vi "Plotting Assemble.vi"(4 "Custom Titles":string[](array[string])=["System Date", "System Time", "Elapsed Time (sec)", "Elapsed Time (hrs)", "Voltage (V)", "RMS Current (Amps)", "Power (Watts)", "Watt Hours (Wh)", "Voltage Total Harmonic Distortion (%)", "Frequency (Hz)", "Apparent Power (VA)", "Power Factor", "TC 1", "TC 2", "TC 3", "TC 4", "TC 5", "TC 6", "TC 7", "TC 8", "TC 9", "TC 10", "TC 11", "TC 12", "TC 13", "TC 14", "TC 15", "TC 16", "TC 17", "TC 18", "TC 19", "TC 20", "TC 21", "TC 22", "TC 23", "TC 24", "TC 25", "TC 26", "TC 27", "TC 28", "TC 29", "TC 30", "AUX 1", "AUX 2", "CAL CL", "Room Setpoint Temperature", "Room Setpoint Humidity", "Room Temperature (°F)", "Room Humidity (%)", "Door Enable", "Room Setpoint Cool Temperature", "Room Setpoint Dehumidification Temperature", "Supply Temperature (°F)", "Cool Temperature (°F)", "Dehumidification Temperature (°F)", "Glycol Temperature (°F)", "Heat Rate (%)", "Steam Rate (%)", "Cool Rate (%)", "Dehumidification Rate (%)", "Room Status", "Room Dry P", "Room Dry I", "Room Humidity P", "Room Humidity I", "Room Heat P", "Room Heat I", "Room Cool Temperature P", "Room Cool Temperature I", "Room Dehumidification Temperature P", "Room Dehumidification Temperature I", "Voltage Setpoint 1", "60 Hz Power", "50 Hz Power", "120V Range", "240V Range", "Ground Line", "Ground Neutral", "Measure Ground Leakage Current", "Room OK", "S1 Freezer Relay", "S1 Cab Relay", "S1 Slide Relay", "Recording Data", "CVS Location", "Point Location"], 6 "Listbox Item Names":string[](array[string])=["System Date", "System Time", "Elapsed Time (sec)", "Elapsed Time (hrs)", "Voltage (V)", "RMS Current (Amps)", "Power (Watts)", "Watt Hours (Wh)", "Voltage Total Harmonic Distortion (%)", "Frequency (Hz)", "Apparent Power (VA)", "Power Factor", "TC 1", "TC 2", "TC 3", "TC 4", "TC 5", "TC 6", "TC 7", "TC 8", "TC 9", "TC 10", "TC 11", "TC 12", "TC 13", "TC 14", "TC 15", "TC 16", "TC 17", "TC 18", "TC 19", "TC 20", "TC 21", "TC 22", "TC 23", "TC 24", "TC 25", "TC 26", "TC 27", "TC 28", "TC 29", "TC 30", "AUX 1", "AUX 2", "CAL CL", "Room Setpoint Temperature", "Room Setpoint Humidity", "Room Temperature (°F)", "Room Humidity (%)", "Door Enable", "Room Setpoint Cool Temperature", "Room Setpoint Dehumidification Temperature", "Supply Temperature (°F)", "Cool Temperature (°F)", "Dehumidification Temperature (°F)", "Glycol Temperature (°F)", "Heat Rate (%)", "Steam Rate (%)", "Cool Rate (%)", "Dehumidification Rate (%)", "Room Status", "Room Dry P", "Room Dry I", "Room Humidity P", "Room Humidity I", "Room Heat P", "Room Heat I", "Room Cool Temperature P", "Room Cool Temperature I", "Room Dehumidification Temperature P", "Room Dehumidification Temperature I", "Voltage Setpoint 1", "60 Hz Power", "50 Hz Power", "120V Range", "240V Range", "Ground Line", "Ground Neutral", "Measure Ground Leakage Current", "Room OK", "S1 Freezer Relay", "S1 Cab Relay", "S1 Slide Relay", "Recording Data", "CVS Location", "Point Location"], 7 "Use Filter?":bool, 8 "Error In":errorcluster, 9 "Full Item Names":string[](array[string])=["System Date", "System Time", "Elapsed Time (sec)", "Elapsed Time (hrs)", "Voltage (V)", "RMS Current (Amps)", "Power (Watts)", "Watt Hours (Wh)", "Voltage Total Harmonic Distortion (%)", "Frequency (Hz)", "Apparent Power (VA)", "Power Factor", "TC 1", "TC 2", "TC 3", "TC 4", "TC 5", "TC 6", "TC 7", "TC 8", "TC 9", "TC 10", "TC 11", "TC 12", "TC 13", "TC 14", "TC 15", "TC 16", "TC 17", "TC 18", "TC 19", "TC 20", "TC 21", "TC 22", "TC 23", "TC 24", "TC 25", "TC 26", "TC 27", "TC 28", "TC 29", "TC 30", "AUX 1", "AUX 2", "CAL CL", "Room Setpoint Temperature", "Room Setpoint Humidity", "Room Temperature (°F)", "Room Humidity (%)", "Door Enable", "Room Setpoint Cool Temperature", "Room Setpoint Dehumidification Temperature", "Supply Temperature (°F)", "Cool Temperature (°F)", "Dehumidification Temperature (°F)", "Glycol Temperature (°F)", "Heat Rate (%)", "Steam Rate (%)", "Cool Rate (%)", "Dehumidification Rate (%)", "Room Status", "Room Dry P", "Room Dry I", "Room Humidity P", "Room Humidity I", "Room Heat P", "Room Heat I", "Room Cool Temperature P", "Room Cool Temperature I", "Room Dehumidification Temperature P", "Room Dehumidification Temperature I", "Voltage Setpoint 1", "60 Hz Power", "50 Hz Power", "120V Range", "240V Range", "Ground Line", "Ground Neutral", "Measure Ground Leakage Current", "Room OK", "S1 Freezer Relay", "S1 Cab Relay", "S1 Slide Relay", "Recording Data", "CVS Location", "Point Location"], 10 "OldVal":i32[](array[numeric]), 11 "All Data":dbl[][](array[numeric])=[[3600091001.703, 12.0, 0.0, 0.0, 115.113976, 0.726104, 73.792992, 3453.956435, 3.4, 59.980007, 83.58474, 0.882852, 7.91, 6.92, 6.4, 327.67, 327.67, 327.67, 327.67, 327.67, 327.67, 327.67, 40.47, 39.09, 39.23, 327.67, 327.67, 327.67, 327.67, 327.67, 327.67, 327.67, 327.67, 327.67, 327.67, 69.95, 327.67, 327.67, 70.08, 327.67, 32767.0, 32767.0, 0.0, 0.0, 1.988, 70.0, 35.0, 69.85, 37.15, 1.0, 55.0, 48.0, 67.6, 55.36, 47.89, 0.0, 38.03, 0.09, 30.61, 7.12, 0.0, 200.0, 15000.0, 400.0, 15000.0, 1000.0, 2000.0, 500.0, 6000.0, 500.0, 6000.0, 115.0, 1.0, 0.0, 1.0, 0.0, 0.0, 1.0, 0.0, 0.0, 0.0, 0.0, 0.0, 0.0, 0.0, 0.0], [3600091002.724, 12.0, 0.0, 0.0, 115.113976, 0.732625, 74.150955, 3453.978342, 3.4, 59.981895, 84.335365, 0.879239, 7.91, 6.92, 6.4, 327.67, 327.67, 327.67, 327.67, 327.67, 327.67, 327.67, 40.47, 39.09, 39.23, 327.67, 327.67, 327.67, 327.67, 327.67, 327.67, 327.67, 327.67, 327.67, 327.67, 69.95, 327.67, 327.67, 70.08, 327.67, 32767.0, 32767.0, 0.001, 0.0, 1.988, 70.0, 35.0, 69.85, 37.15, 1.0, 55.0, 48.0, 67.6, 55.36, 47.89, 0.0, 38.03, 0.09, 30.61, 7.12, 0.0, 200.0, 15000.0, 400.0, 15000.0, 1000.0, 2000.0, 500.0, 6000.0, 500.0, 6000.0, 115.0, 1.0, 0.0, 1.0, 0.0, 0.0, 1.0, 0.0, 0.0, 0.0, 0.0, 0.0, 0.0, 0.0, 0.0], [3600091003.749, 12.0, 0.0, 0.0, 115.094734, 0.72875, 73.917732, 3454.000256, 3.4, 59.980373, 84.227455, 0.878872, 7.88, 6.92, 6.4, 327.67, 327.67, 327.67, 327.67, 327.67, 327.67, 327.67, 40.47, 39.09, 39.23, 327.67, 327.67, 327.67, 327.67, 327.67, 327.67, 327.67, 327.67, 327.67, 327.67, 70.0, 327.67, 327.67, 70.14, 327.67, 32767.0, 32767.0, 0.001, 0.0, 1.988, 70.0, 35.0, 69.85, 37.15, 1.0, 55.0, 48.0, 67.6, 55.36, 47.89, 0.0, 38.03, 0.09, 30.61, 7.12, 0.0, 200.0, 15000.0, 400.0, 15000.0, 1000.0, 2000.0, 500.0, 6000.0, 500.0, 6000.0, 115.0, 1.0, 0.0, 1.0, 0.0, 0.0, 1.0, 0.0, 0.0, 0.0, 0.0, 0.0, 0.0, 0.0, 0.0], [3600091004.771, 12.0, 0.0, 0.0, 115.123596, 0.731687, 73.960884, 3454.019387, 3.2, 59.983654, 84.234489, 0.878036, 7.88, 6.92, 6.4, 327.67, 327.67, 327.67, 327.67, 327.67, 327.67, 327.67, 40.47, 39.09, 39.23, 327.67, 327.67, 327.67, 327.67, 327.67, 327.67, 327.67, 327.67, 327.67, 327.67, 70.0, 327.67, 327.67, 70.14, 327.67, 32767.0, 32767.0, 0.001, 0.0, 1.987, 70.0, 35.0, 69.85, 37.15, 1.0, 55.0, 48.0, 67.6, 55.36, 47.89, 0.0, 38.02, 0.09, 30.61, 7.12, 0.0, 200.0, 15000.0, 400.0, 15000.0, 1000.0, 2000.0, 500.0, 6000.0, 500.0, 6000.0, 115.0, 1.0, 0.0, 1.0, 0.0, 0.0, 1.0, 0.0, 0.0, 0.0, 0.0, 0.0, 0.0, 0.0, 0.0], [3600091005.799, 12.0, 0.0, 0.0, 115.113976, 0.72825, 73.662361, 3454.041219, 3.4, 59.985176, 83.831749, 0.878693, 7.88, 6.92, 6.4, 327.67, 327.67, 327.67, 327.67, 327.67, 327.67, 327.67, 40.44, 39.04, 39.23, 327.67, 327.67, 327.67, 327.67, 327.67, 327.67, 327.67, 327.67, 327.67, 327.67, 70.0, 327.67, 327.67, 70.14, 327.67, 32767.0, 32767.0, 0.001, 0.0, 1.987, 70.0, 35.0, 69.85, 37.15, 1.0, 55.0, 48.0, 67.6, 55.36, 47.89, 0.0, 38.02, 0.09, 30.61, 7.12, 0.0, 200.0, 15000.0, 400.0, 15000.0, 1000.0, 2000.0, 500.0, 6000.0, 500.0, 6000.0, 115.0, 1.0, 0.0, 1.0, 0.0, 0.0, 1.0, 0.0, 0.0, 0.0, 0.0, 0.0, 0.0, 0.0, 0.0], [3600091006.815, 12.0, 0.0, 0.0, 115.123596, 0.725771, 73.487831, 3454.063036, 3.4, 59.986942, 83.553345, 0.879532, 7.88, 6.92, 6.4, 327.67, 327.67, 327.67, 327.67, 327.67, 327.67, 327.67, 40.44, 39.04, 39.23, 327.67, 327.67, 327.67, 327.67, 327.67, 327.67, 327.67, 327.67, 327.67, 327.67, 70.0, 327.67, 327.67, 70.14, 327.67, 32767.0, 32767.0, 0.001, 0.0, 1.988, 70.0, 35.0, 69.85, 37.15, 1.0, 55.0, 48.0, 67.6, 55.36, 47.89, 0.0, 38.02, 0.08, 30.61, 7.12, 0.0, 200.0, 15000.0, 400.0, 15000.0, 1000.0, 2000.0, 500.0, 6000.0, 500.0, 6000.0, 115.0, 1.0, 0.0, 1.0, 0.0, 0.0, 1.0, 0.0, 0.0, 0.0, 0.0, 0.0, 0.0, 0.0, 0.0], [3600091007.834, 12.0, 0.0, 0.0, 115.104355, 0.728729, 73.744789, 3454.082127, 3.4, 59.984016, 83.879898, 0.879171, 7.88, 6.92, 6.4, 327.67, 327.67, 327.67, 327.67, 327.67, 327.67, 327.67, 40.44, 39.04, 39.23, 327.67, 327.67, 327.67, 327.67, 327.67, 327.67, 327.67, 327.67, 327.67, 327.67, 70.0, 327.67, 327.67, 70.14, 327.67, 32767.0, 32767.0, 0.001, 0.0, 1.988, 70.0, 35.0, 69.85, 37.15, 1.0, 55.0, 48.0, 67.6, 55.36, 47.89, 0.0, 38.02, 0.08, 30.61, 7.12, 0.0, 200.0, 15000.0, 400.0, 15000.0, 1000.0, 2000.0, 500.0, 6000.0, 500.0, 6000.0, 115.0, 1.0, 0.0, 1.0, 0.0, 0.0, 1.0, 0.0, 0.0, 0.0, 0.0, 0.0, 0.0, 0.0, 0.0], [3600091008.851, 12.0, 0.0, 0.0, 115.123596, 0.726167, 73.607307, 3454.103967, 3.3, 59.985229, 83.598915, 0.880482, 7.88, 6.92, 6.4, 327.67, 327.67, 327.67, 327.67, 327.67, 327.67, 327.67, 40.44, 39.04, 39.23, 327.67, 327.67, 327.67, 327.67, 327.67, 327.67, 327.67, 327.67, 327.67, 327.67, 70.0, 327.67, 327.67, 70.14, 327.67, 32767.0, 32767.0, 0.001, 0.001, 1.988, 70.0, 35.0, 69.85, 37.15, 1.0, 55.0, 48.0, 67.6, 55.36, 47.89, 0.0, 38.02, 0.08, 30.61, 7.12, 0.0, 200.0, 15000.0, 400.0, 15000.0, 1000.0, 2000.0, 500.0, 6000.0, 500.0, 6000.0, 115.0, 1.0, 0.0, 1.0, 0.0, 0.0, 1.0, 0.0, 0.0, 0.0, 0.0, 0.0, 0.0, 0.0, 0.0], [3600091009.874, 12.0, 0.0, 0.0, 115.113976, 0.728542, 73.781647, 3454.123084, 3.4, 59.985569, 83.865326, 0.879763, 7.88, 6.87, 6.4, 327.67, 327.67, 327.67, 327.67, 327.67, 327.67, 327.67, 40.47, 39.04, 39.23, 327.67, 327.67, 327.67, 327.67, 327.67, 327.67, 327.67, 327.67, 327.67, 327.67, 70.0, 327.67, 327.67, 70.14, 327.67, 32767.0, 32767.0, 0.001, 0.001, 1.988, 70.0, 35.0, 69.85, 37.15, 1.0, 55.0, 48.0, 67.6, 55.36, 47.89, 0.0, 38.01, 0.08, 30.61, 7.12, 0.0, 200.0, 15000.0, 400.0, 15000.0, 1000.0, 2000.0, 500.0, 6000.0, 500.0, 6000.0, 115.0, 1.0, 0.0, 1.0, 0.0, 0.0, 1.0, 0.0, 0.0, 0.0, 0.0, 0.0, 0.0, 0.0, 0.0], [3600091010.892, 12.0, 0.0, 0.0, 115.104355, 0.725438, 73.578506, 3454.144929, 3.3, 59.984901, 83.501015, 0.881169, 7.88, 6.87, 6.4, 327.67, 327.67, 327.67, 327.67, 327.67, 327.67, 327.67, 40.47, 39.04, 39.23, 327.67, 327.67, 327.67, 327.67, 327.67, 327.67, 327.67, 327.67, 327.67, 327.67, 70.0, 327.67, 327.67, 70.14, 327.67, 32767.0, 32767.0, 0.001, 0.001, 1.988, 70.0, 35.0, 69.85, 37.15, 1.0, 55.0, 48.0, 67.6, 55.36, 47.89, 0.0, 38.01, 0.08, 30.61, 7.12, 0.0, 200.0, 15000.0, 400.0, 15000.0, 1000.0, 2000.0, 500.0, 6000.0, 500.0, 6000.0, 115.0, 1.0, 0.0, 1.0, 0.0, 0.0, 1.0, 0.0, 0.0, 0.0, 0.0, 0.0, 0.0, 0.0, 0.0], [3600091011.915, 12.0, 0.0, 0.0, 115.104355, 0.722, 73.502365, 3454.16674, 3.4, 59.98167, 83.105339, 0.884448, 7.83, 6.87, 6.4, 327.67, 327.67, 327.67, 327.67, 327.67, 327.67, 327.67, 40.44, 39.04, 39.23, 327.67, 327.67, 327.67, 327.67, 327.67, 327.67, 327.67, 327.67, 327.67, 327.67, 69.92, 327.67, 327.67, 70.08, 327.67, 32767.0, 32767.0, 0.001, 0.001, 1.988, 70.0, 35.0, 69.85, 37.15, 1.0, 55.0, 48.0, 67.6, 55.36, 47.89, 0.0, 38.01, 0.08, 30.61, 7.12, 0.0, 200.0, 15000.0, 400.0, 15000.0, 1000.0, 2000.0, 500.0, 6000.0, 500.0, 6000.0, 115.0, 1.0, 0.0, 1.0, 0.0, 0.0, 1.0, 0.0, 0.0, 0.0, 0.0, 0.0, 0.0, 0.0, 0.0], [3600091012.934, 12.0, 0.0, 0.0, 115.094727, 0.723542, 73.421265, 3454.185795, 3.4, 59.981655, 83.275833, 0.881664, 7.83, 6.87, 6.4, 327.67, 327.67, 327.67, 327.67, 327.67, 327.67, 327.67, 40.44, 39.04, 39.23, 327.67, 327.67, 327.67, 327.67, 327.67, 327.67, 327.67, 327.67, 327.67, 327.67, 69.92, 327.67, 327.67, 70.08, 327.67, 32767.0, 32767.0, 0.001, 0.0, 1.988, 70.0, 35.0, 69.85, 37.15, 1.0, 55.0, 48.0, 67.6, 55.36, 47.89, 0.0, 38.01, 0.07, 30.62, 7.12, 0.0, 200.0, 15000.0, 400.0, 15000.0, 1000.0, 2000.0, 500.0, 6000.0, 500.0, 6000.0, 115.0, 1.0, 0.0, 1.0, 0.0, 0.0, 1.0, 0.0, 0.0, 0.0, 0.0, 0.0, 0.0, 0.0, 0.0], [3600091013.956, 12.0, 0.0, 0.0, 115.113976, 0.721937, 73.541336, 3454.207582, 3.3, 59.98288, 83.105095, 0.88492, 7.83, 6.87, 6.4, 327.67, 327.67, 327.67, 327.67, 327.67, 327.67, 327.67, 40.44, 39.04, 39.23, 327.67, 327.67, 327.67, 327.67, 327.67, 327.67, 327.67, 327.67, 327.67, 327.67, 70.0, 327.67, 327.67, 70.14, 327.67, 32767.0, 32767.0, 0.001, 0.0, 1.988, 70.0, 35.0, 69.85, 37.15, 1.0, 55.0, 48.0, 67.33, 55.36, 47.89, 0.0, 38.0, 0.07, 30.62, 7.12, 0.0, 200.0, 15000.0, 400.0, 15000.0, 1000.0, 2000.0, 500.0, 6000.0, 500.0, 6000.0, 115.0, 1.0, 0.0, 1.0, 0.0, 0.0, 1.0, 0.0, 0.0, 0.0, 0.0, 0.0, 0.0, 0.0, 0.0], [3600091014.973, 12.0, 0.0, 0.0, 115.133224, 0.725083, 73.722015, 3454.229415, 3.4, 59.983387, 83.481186, 0.883097, 7.83, 6.87, 6.4, 327.67, 327.67, 327.67, 327.67, 327.67, 327.67, 327.67, 40.44, 39.04, 39.23, 327.67, 327.67, 327.67, 327.67, 327.67, 327.67, 327.67, 327.67, 327.67, 327.67, 70.0, 327.67, 327.67, 70.14, 327.67, 32767.0, 32767.0, 0.001, 0.0, 1.988, 70.0, 35.0, 69.85, 37.15, 1.0, 55.0, 48.0, 67.33, 55.36, 47.89, 0.0, 39.04, 0.07, 30.62, 7.12, 0.0, 200.0, 15000.0, 400.0, 15000.0, 1000.0, 2000.0, 500.0, 6000.0, 500.0, 6000.0, 115.0, 1.0, 0.0, 1.0, 0.0, 0.0, 1.0, 0.0, 0.0, 0.0, 0.0, 0.0, 0.0, 0.0, 0.0], [3600091015.997, 12.0, 0.0, 0.0, 115.094727, 0.722229, 73.60537, 3454.24855, 3.3, 59.983395, 83.124771, 0.885481, 7.83, 6.87, 6.4, 327.67, 327.67, 327.67, 327.67, 327.67, 327.67, 327.67, 40.44, 39.04, 39.23, 327.67, 327.67, 327.67, 327.67, 327.67, 327.67, 327.67, 327.67, 327.67, 327.67, 70.0, 327.67, 327.67, 70.14, 327.67, 32767.0, 32767.0, 0.001, 0.0, 1.988, 70.0, 35.0, 69.85, 37.15, 1.0, 55.0, 48.0, 67.33, 55.36, 47.89, 0.0, 39.04, 0.07, 30.62, 7.12, 0.0, 200.0, 15000.0, 400.0, 15000.0, 1000.0, 2000.0, 500.0, 6000.0, 500.0, 6000.0, 115.0, 1.0, 0.0, 1.0, 0.0, 0.0, 1.0, 0.0, 0.0, 0.0, 0.0, 0.0, 0.0, 0.0, 0.0], [3600091017.018, 12.0, 0.0, 0.0, 115.142845, 0.728646, 73.968193, 3454.270419, 3.2, 59.984619, 83.898354, 0.881641, 7.83, 6.87, 6.35, 327.67, 327.67, 327.67, 327.67, 327.67, 327.67, 327.67, 40.44, 39.04, 39.23, 327.67, 327.67, 327.67, 327.67, 327.67, 327.67, 327.67, 327.67, 327.67, 327.67, 70.0, 327.67, 327.67, 70.14, 327.67, 32767.0, 32767.0, 0.001, 0.001, 1.988, 70.0, 35.0, 69.85, 37.15, 1.0, 55.0, 48.0, 67.33, 55.36, 47.89, 0.0, 39.04, 0.07, 30.62, 7.12, 0.0, 200.0, 15000.0, 400.0, 15000.0, 1000.0, 2000.0, 500.0, 6000.0, 500.0, 6000.0, 115.0, 1.0, 0.0, 1.0, 0.0, 0.0, 1.0, 0.0, 0.0, 0.0, 0.0, 0.0, 0.0, 0.0, 0.0], [3600091018.039, 12.0, 0.0, 0.0, 115.104355, 0.73125, 73.90947, 3454.292285, 3.3, 59.98568, 84.170059, 0.878097, 7.83, 6.87, 6.35, 327.67, 327.67, 327.67, 327.67, 327.67, 327.67, 327.67, 40.44, 39.04, 39.23, 327.67, 327.67, 327.67, 327.67, 327.67, 327.67, 327.67, 327.67, 327.67, 327.67, 69.95, 327.67, 327.67, 70.08, 327.67, 32767.0, 32767.0, 0.001, 0.001, 1.988, 70.0, 35.0, 69.85, 37.15, 1.0, 55.0, 48.0, 67.33, 55.36, 47.89, 0.0, 39.05, 0.07, 30.62, 7.12, 0.0, 200.0, 15000.0, 400.0, 15000.0, 1000.0, 2000.0, 500.0, 6000.0, 500.0, 6000.0, 115.0, 1.0, 0.0, 1.0, 0.0, 0.0, 1.0, 0.0, 0.0, 0.0, 0.0, 0.0, 0.0, 0.0, 0.0], [3600091019.059, 12.0, 0.0, 0.0, 115.104355, 0.727896, 73.668884, 3454.311388, 3.3, 59.986122, 83.783981, 0.879272, 7.83, 6.87, 6.4, 327.67, 327.67, 327.67, 327.67, 327.67, 327.67, 327.67, 40.44, 39.04, 39.23, 327.67, 327.67, 327.67, 327.67, 327.67, 327.67, 327.67, 327.67, 327.67, 327.67, 69.95, 327.67, 327.67, 70.08, 327.67, 32767.0, 32767.0, 0.001, 0.001, 1.988, 70.0, 35.0, 69.85, 37.15, 1.0, 55.0, 48.0, 67.33, 55.36, 47.89, 0.0, 39.05, 0.07, 30.62, 7.12, 0.0, 200.0, 15000.0, 400.0, 15000.0, 1000.0, 2000.0, 500.0, 6000.0, 500.0, 6000.0, 115.0, 1.0, 0.0, 1.0, 0.0, 0.0, 1.0, 0.0, 0.0, 0.0, 0.0, 0.0, 0.0, 0.0, 0.0], [3600091020.076, 12.0, 0.0, 0.0, 115.113976, 0.729708, 73.698441, 3454.333193, 3.3, 59.986202, 83.999626, 0.877366, 7.83, 6.87, 6.4, 327.67, 327.67, 327.67, 327.67, 327.67, 327.67, 327.67, 40.44, 39.04, 39.23, 327.67, 327.67, 327.67, 327.67, 327.67, 327.67, 327.67, 327.67, 327.67, 327.67, 69.95, 327.67, 327.67, 70.08, 327.67, 32767.0, 32767.0, 0.001, 0.001, 1.988, 70.0, 35.0, 69.85, 37.15, 1.0, 55.0, 48.0, 67.33, 55.36, 47.89, 0.0, 39.05, 0.06, 30.62, 7.12, 0.0, 200.0, 15000.0, 400.0, 15000.0, 1000.0, 2000.0, 500.0, 6000.0, 500.0, 6000.0, 115.0, 1.0, 0.0, 1.0, 0.0, 0.0, 1.0, 0.0, 0.0, 0.0, 0.0, 0.0, 0.0, 0.0, 0.0]] format="%.6f") -> (0 "Error Out":errorcluster, 3 "Mixed Signal Graph":T1(graph))   [LabVIEW 2016]
panel:
  out "time stamp":timestamp
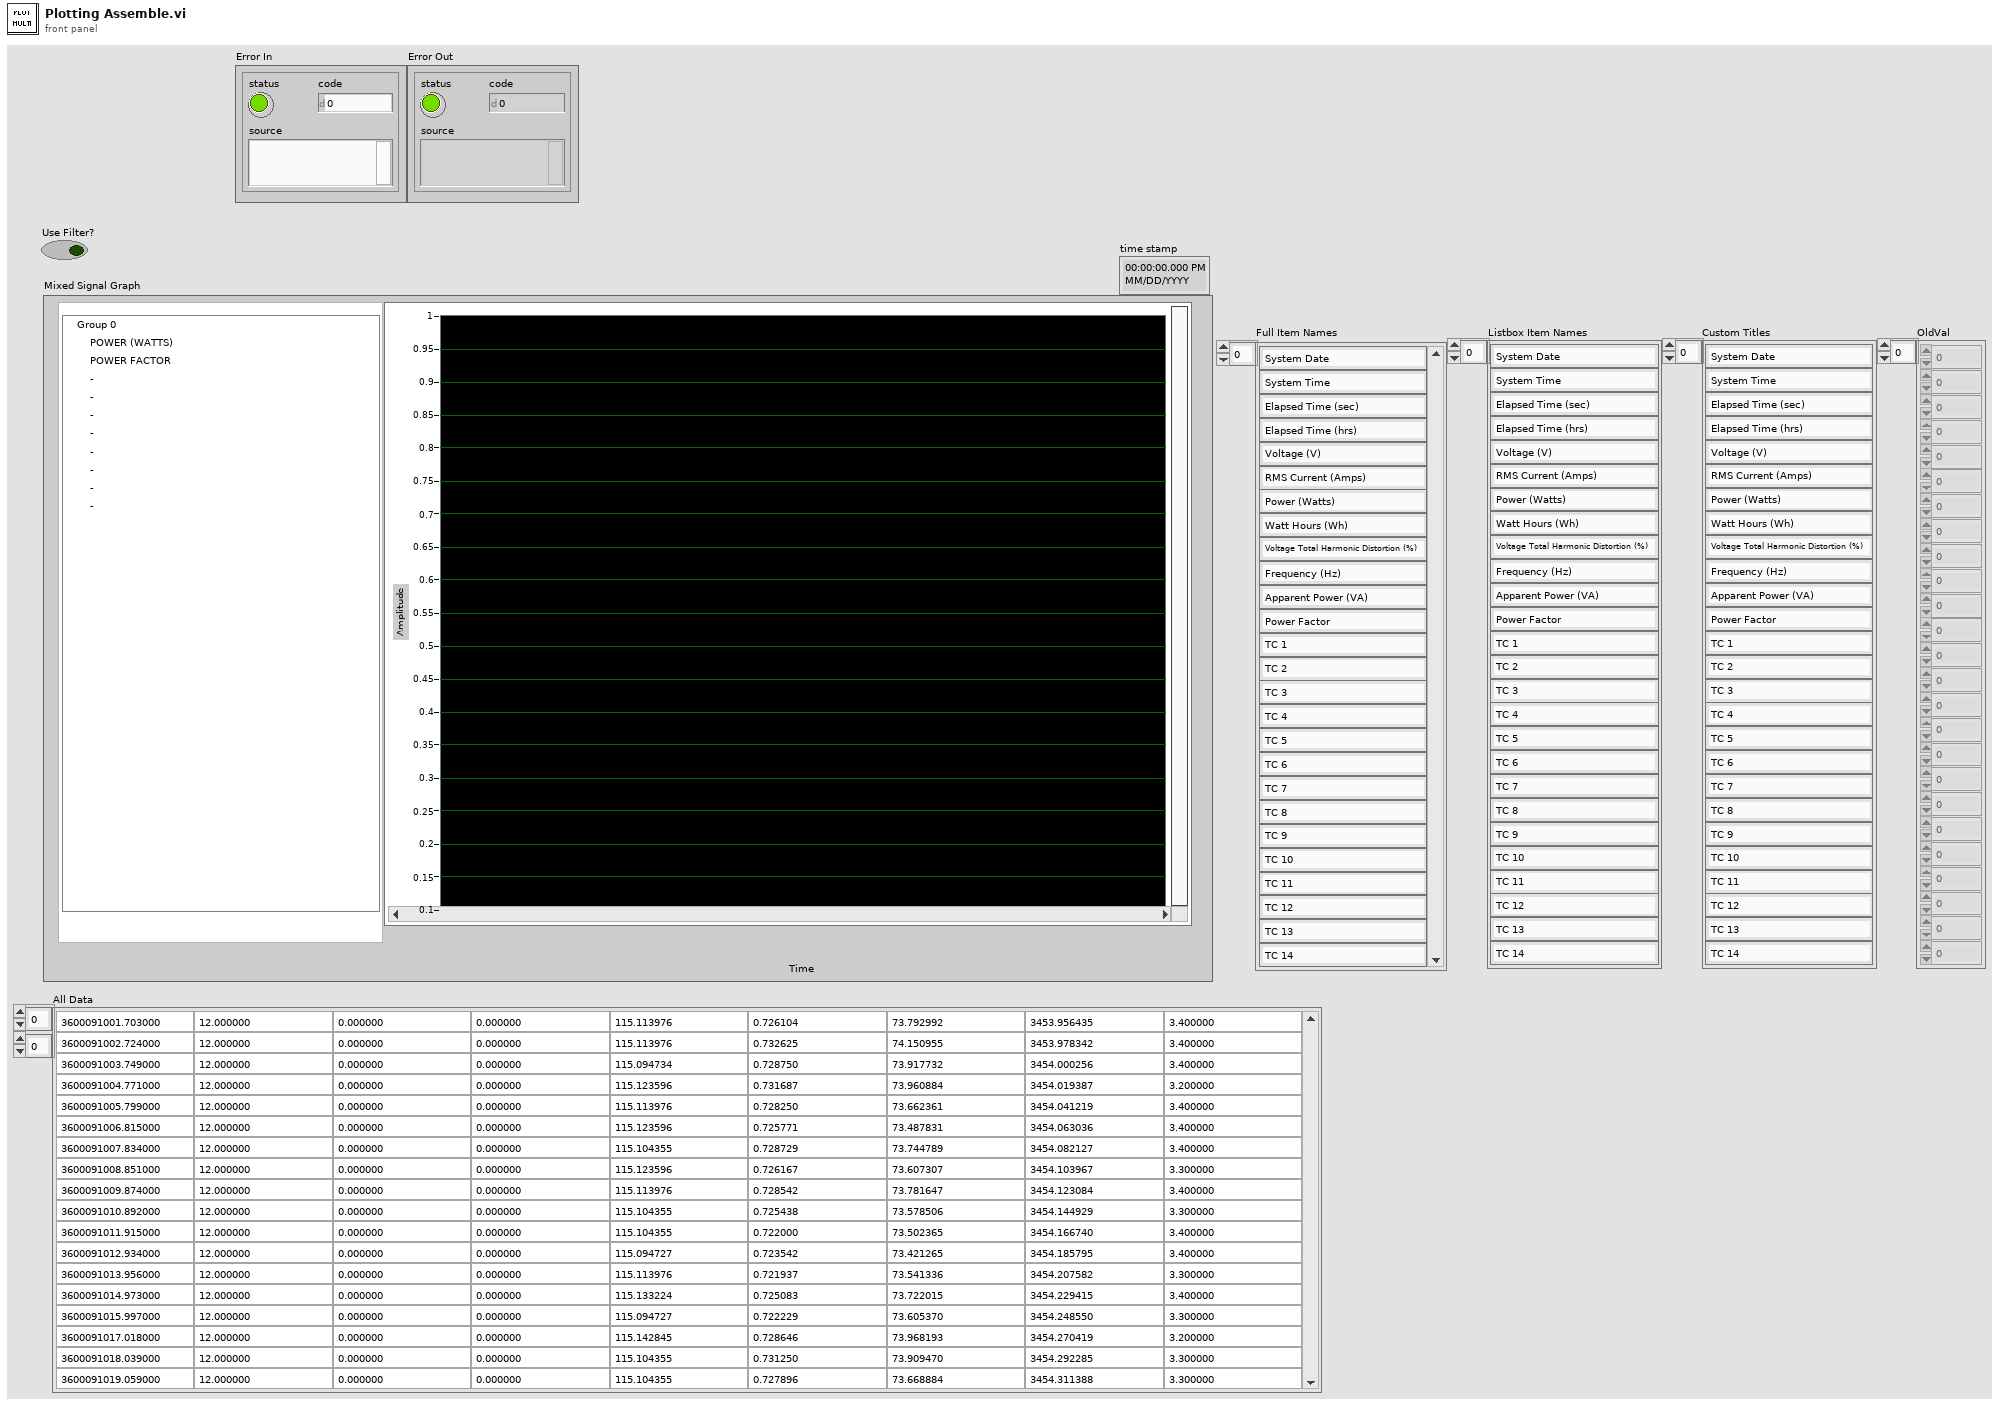
[diagram p1: front panel]
types:
  T1 = cluster{"Waveform Graph":waveform(dbl), "Waveform Graph":waveform(dbl), "Waveform Graph":waveform(dbl), "Waveform Graph":waveform(dbl), "Waveform Graph":waveform(dbl), "Waveform Graph":waveform(dbl), "Waveform Graph":waveform(dbl), "Waveform Graph":waveform(dbl), "Waveform Graph":waveform(dbl), "Waveform Graph":waveform(dbl)}
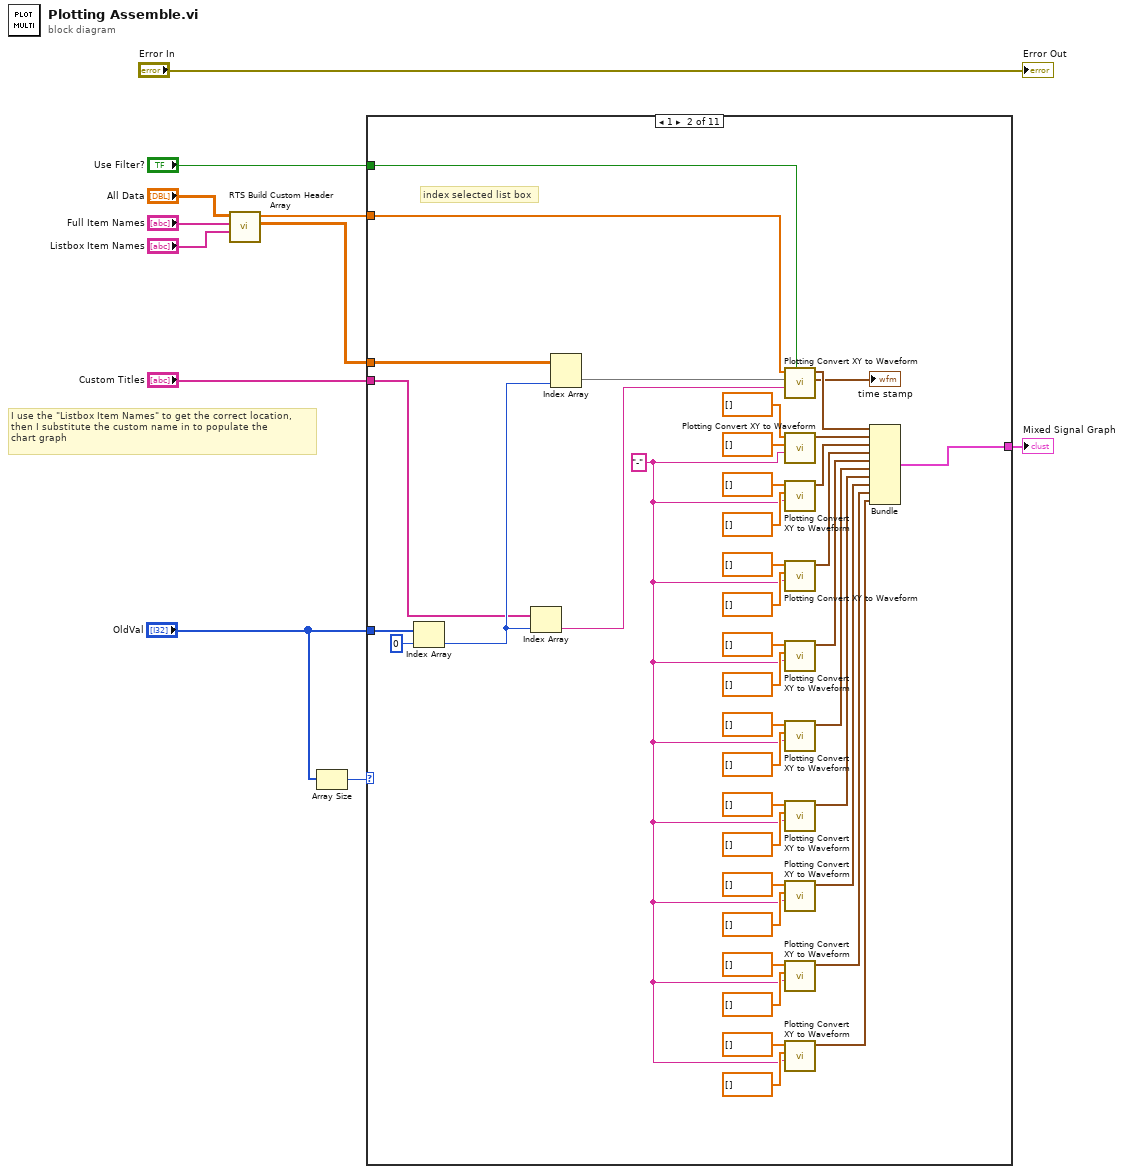
[diagram p0: block diagram]
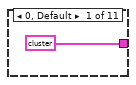
[diagram p2: hidden frame]
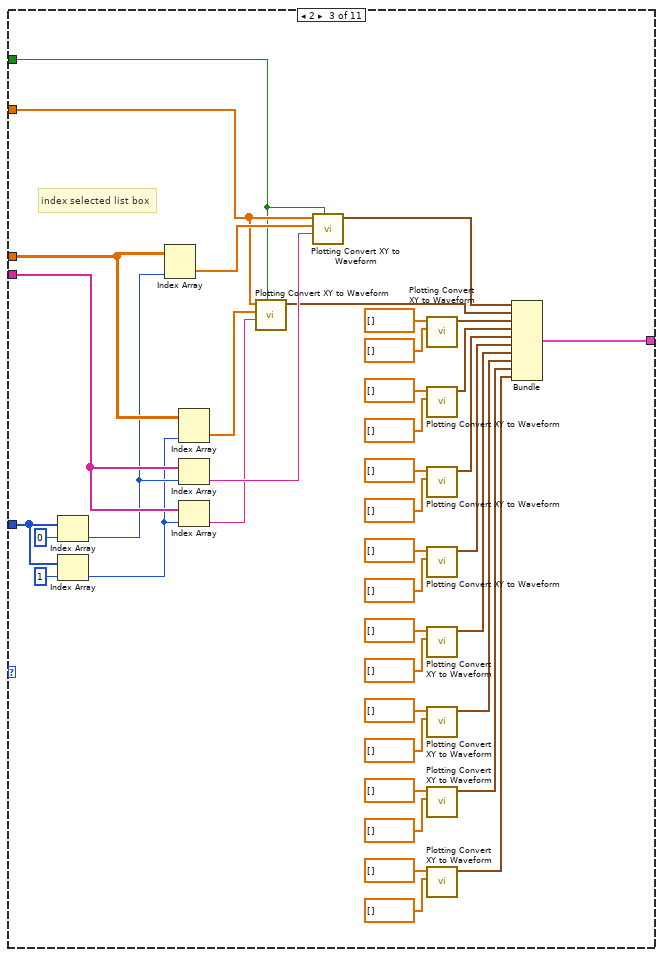
[diagram p3: hidden frame]
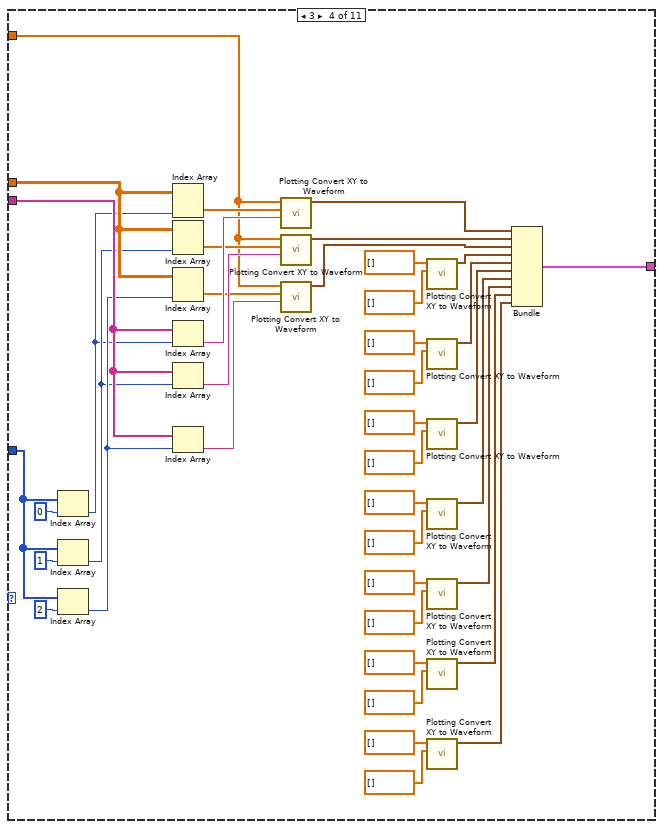
[diagram p4: hidden frame]
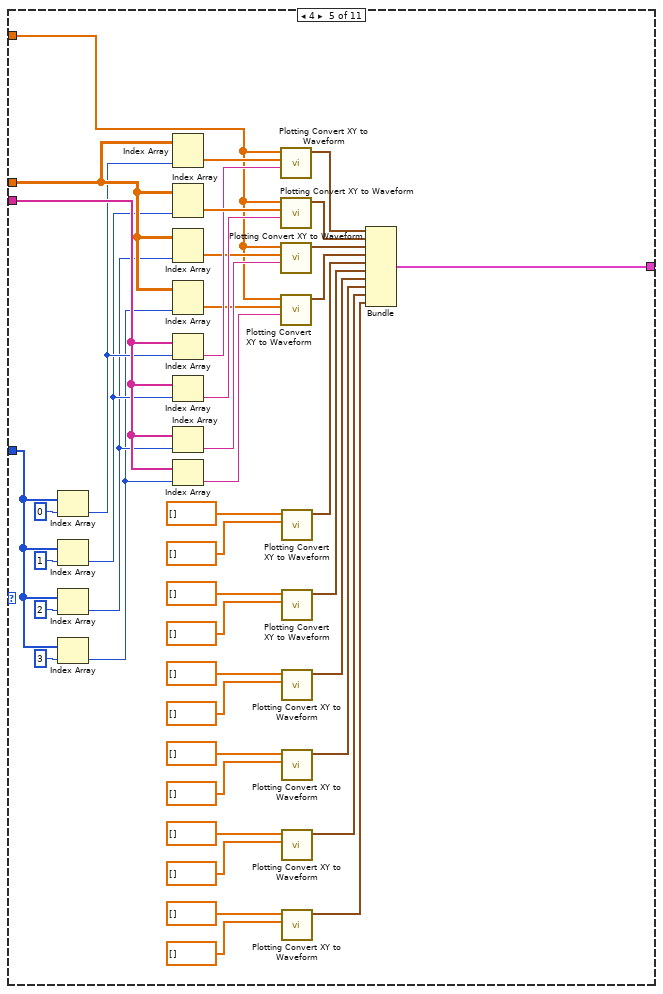
[diagram p5: hidden frame]
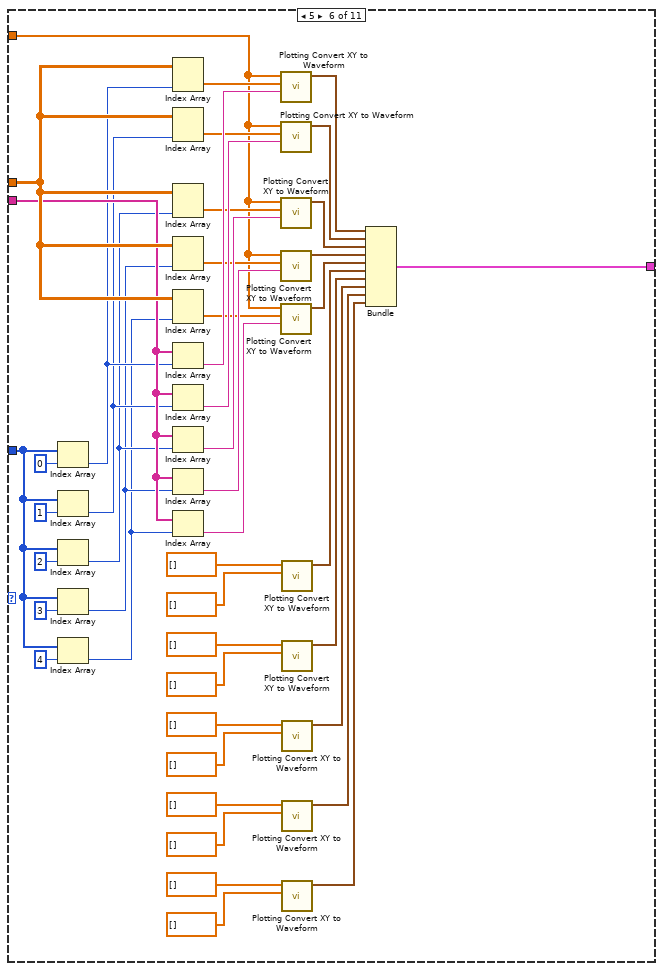
[diagram p6: hidden frame]
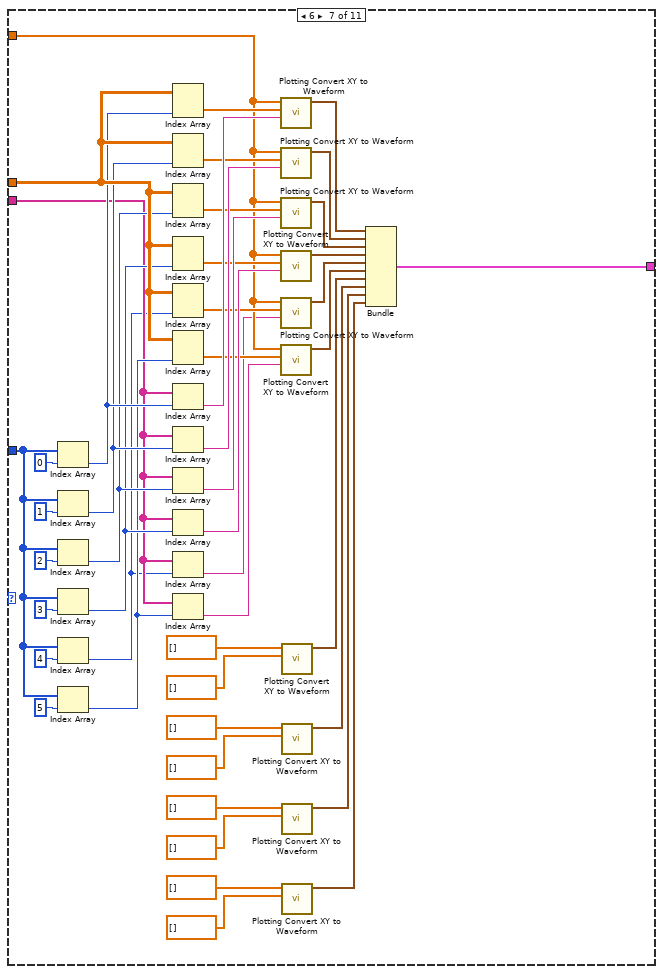
[diagram p7: hidden frame]
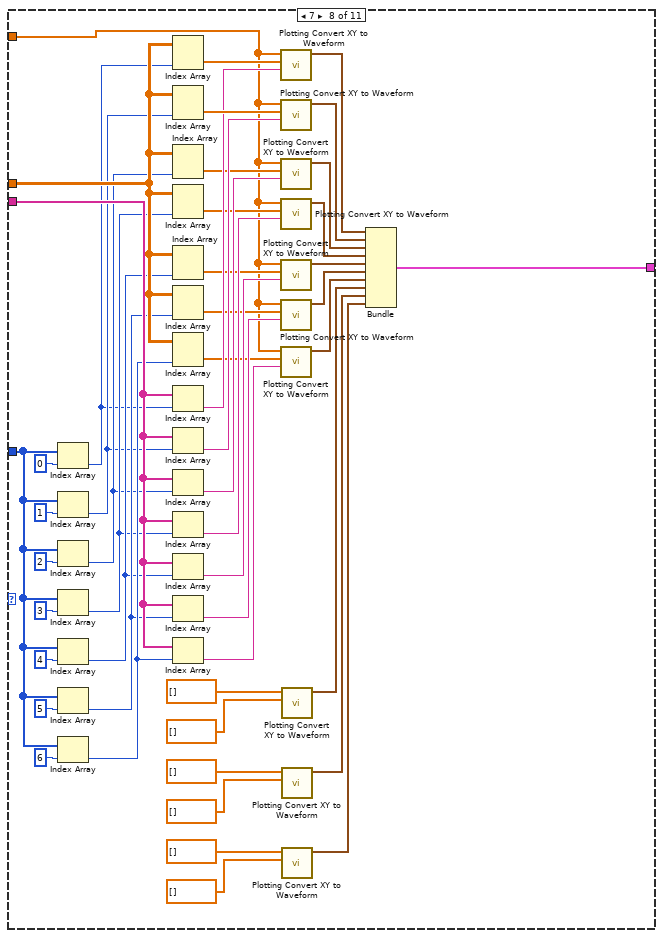
[diagram p8: hidden frame]
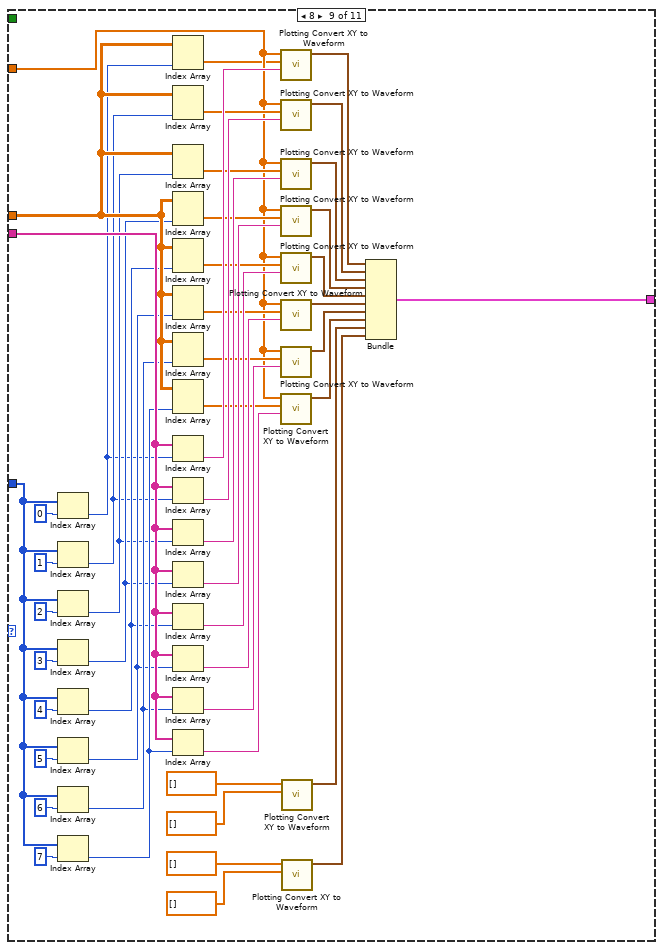
[diagram p9: hidden frame]
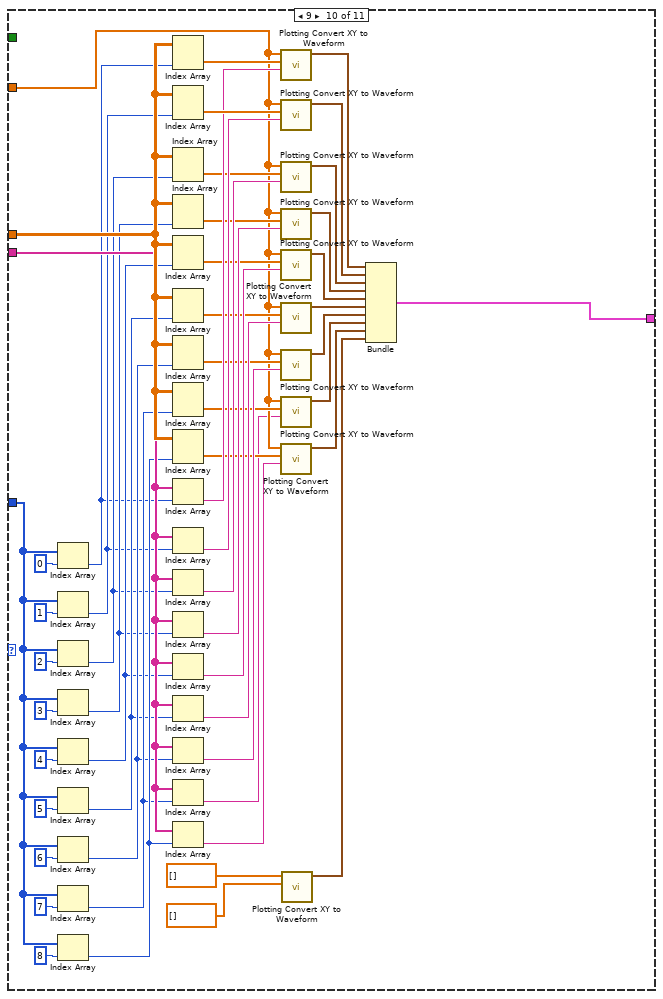
[diagram p10: hidden frame]
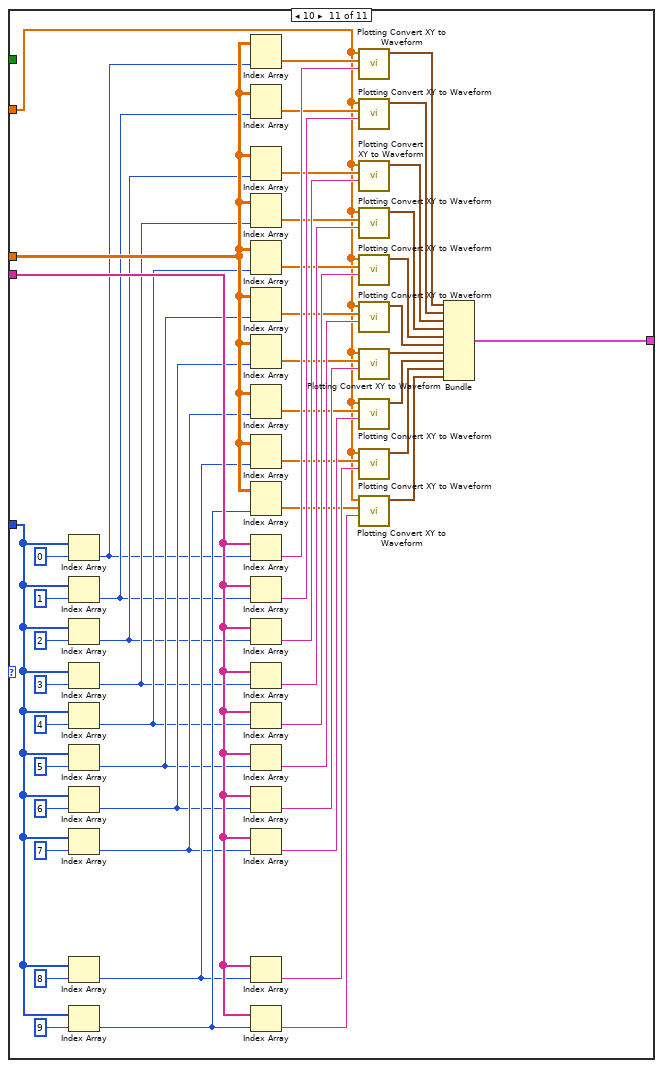
[diagram p11: hidden frame]
diagram:
  # "I use the \"Listbox Item Names\" to get the correct location,\nthen I substitute the custom name in to populate the \nchart graph"
  n1 = call "RTS Build Custom Header Array.vi"("Listbox Item Names in"="Listbox Item Names", "Full Item Names"="Full Item Names", "All Data in"="All Data") -> ("Parsed Array"=w5:dbl[][], "Time Data"=w6:dbl[])  [unwired: 4 in, 3 out]
  n2 = Array Size(array="OldVal") -> (size(s)=w11:i32)
  n3 = case shown="1" w11 {
    tunnel: w5 -> [_ w51 w91 w132 w175 w219 w265 w316 w366 w420 w476]
    tunnel: [T1 {"Waveform Graph"={"t0"=timestamp(0 s since 1904-01-01), "dt"=1.0, "Y"=[]}, "Waveform Graph"={"t0"=timestamp(0 s since 1904-01-01), "dt"=1.0, "Y"=[]}, "Waveform Graph"={"t0"=timestamp(0 s since 1904-01-01), "dt"=1.0, "Y"=[]}, "Waveform Graph"={"t0"=timestamp(0 s since 1904-01-01), "dt"=1.0, "Y"=[]}, "Waveform Graph"={"t0"=timestamp(0 s since 1904-01-01), "dt"=1.0, "Y"=[]}, "Waveform Graph"={"t0"=timestamp(0 s since 1904-01-01), "dt"=1.0, "Y"=[]}, "Waveform Graph"={"t0"=timestamp(0 s since 1904-01-01), "dt"=1.0, "Y"=[]}, "Waveform Graph"={"t0"=timestamp(0 s since 1904-01-01), "dt"=1.0, "Y"=[]}, "Waveform Graph"={"t0"=timestamp(0 s since 1904-01-01), "dt"=1.0, "Y"=[]}, "Waveform Graph"={"t0"=timestamp(0 s since 1904-01-01), "dt"=1.0, "Y"=[]}} w50 w92 w131 w174 w221 w267 w315 w368 w419 w432] -> w10
    tunnel: "OldVal" -> [_ w49 w90 w133 w176 w220 w266 w317 w367 w421 w473]
    tunnel: w6 -> [_ w17 w85 w122 w161 w202 w246 w290 w319 w388 w436]
    tunnel: "Custom Titles" -> [_ w19 w82 w119 w158 w199 w224 w287 w335 w385 w437]
    tunnel: "Use Filter?" -> [_ w13 w53 _ _ _ _ _ _ _ _]
    frame 0, Default {
    }
    frame 1 {
      w14 = "-" ("Plot Name")
      # "index selected list box"
      n4 = Index Array(array=w49, index=0) -> (element=w20:i32)
      n5 = Index Array(array=w19, index=w20) -> (element=w18:string)
      n6 = Index Array(array=w51, index (col)=w20) -> (element=w16:dbl[])  [unwired: 1 in]
      n7 = call "Plotting Convert XY to Waveform.vi"("Use Filter?"=w13, "Plot Name"=w18, "Y"=w16, "X"=w17) -> ("time stamp"=→"time stamp":timestamp, "Waveform Graph"=w48:waveform(dbl))  [unwired: 5 in, 1 out]
      n8 = call "Plotting Convert XY to Waveform.vi"("Plot Name"=w14, "Y"=dbl[] [], "X"=dbl[] []) -> ("Waveform Graph"=w45:waveform(dbl))  [unwired: 6 in, 2 out]
      n9 = call "Plotting Convert XY to Waveform.vi"("Plot Name"=w14, "Y"=dbl[] [], "X"=dbl[] []) -> ("Waveform Graph"=w42:waveform(dbl))  [unwired: 6 in, 2 out]
      n10 = call "Plotting Convert XY to Waveform.vi"("Plot Name"=w14, "Y"=dbl[] [], "X"=dbl[] []) -> ("Waveform Graph"=w39:waveform(dbl))  [unwired: 6 in, 2 out]
      n11 = call "Plotting Convert XY to Waveform.vi"("Plot Name"=w14, "Y"=dbl[] [], "X"=dbl[] []) -> ("Waveform Graph"=w36:waveform(dbl))  [unwired: 6 in, 2 out]
      n12 = call "Plotting Convert XY to Waveform.vi"("Plot Name"=w14, "Y"=dbl[] [], "X"=dbl[] []) -> ("Waveform Graph"=w33:waveform(dbl))  [unwired: 6 in, 2 out]
      n13 = call "Plotting Convert XY to Waveform.vi"("Plot Name"=w14, "Y"=dbl[] [], "X"=dbl[] []) -> ("Waveform Graph"=w30:waveform(dbl))  [unwired: 6 in, 2 out]
      n14 = call "Plotting Convert XY to Waveform.vi"("Plot Name"=w14, "Y"=dbl[] [], "X"=dbl[] []) -> ("Waveform Graph"=w27:waveform(dbl))  [unwired: 6 in, 2 out]
      n15 = call "Plotting Convert XY to Waveform.vi"("Plot Name"=w14, "Y"=dbl[] [], "X"=dbl[] []) -> ("Waveform Graph"=w24:waveform(dbl))  [unwired: 6 in, 2 out]
      n16 = call "Plotting Convert XY to Waveform.vi"("Plot Name"=w14, "Y"=dbl[] [], "X"=dbl[] []) -> ("Waveform Graph"=w21:waveform(dbl))  [unwired: 6 in, 2 out]
      n17 = Bundle "Bundle"("Waveform Graph"=w48, "Waveform Graph"=w45, "Waveform Graph"=w42, "Waveform Graph"=w39, "Waveform Graph"=w36, "Waveform Graph"=w33, "Waveform Graph"=w30, "Waveform Graph"=w27, "Waveform Graph"=w24, "Waveform Graph"=w21) -> (w50:T1)  [unwired: 1 in]
    }
    frame 2 {
      # "index selected list box"
      n18 = Index Array(array=w90, index=0) -> (element=w55:i32)
      n19 = Index Array(array=w90, index=1) -> (element=w54:i32)
      n20 = Index Array(array=w91, index (col)=w55) -> (element=w89:dbl[])  [unwired: 1 in]
      n21 = Index Array(array=w91, index (col)=w54) -> (element=w84:dbl[])  [unwired: 1 in]
      n22 = Index Array(array=w82, index=w55) -> (element=w86:string)
      n23 = Index Array(array=w82, index=w54) -> (element=w80:string)
      n24 = call "Plotting Convert XY to Waveform.vi"("Use Filter?"=w53, "Plot Name"=w80, "Y"=w84, "X"=w85) -> ("Waveform Graph"=w83:waveform(dbl))  [unwired: 5 in, 2 out]
      n25 = call "Plotting Convert XY to Waveform.vi"("Use Filter?"=w53, "Plot Name"=w86, "Y"=w89, "X"=w85) -> ("Waveform Graph"=w88:waveform(dbl))  [unwired: 5 in, 2 out]
      n26 = call "Plotting Convert XY to Waveform.vi"("Y"=dbl[] [], "X"=dbl[] []) -> ("Waveform Graph"=w77:waveform(dbl))  [unwired: 7 in, 2 out]
      n27 = call "Plotting Convert XY to Waveform.vi"("Y"=dbl[] [], "X"=dbl[] []) -> ("Waveform Graph"=w74:waveform(dbl))  [unwired: 7 in, 2 out]
      n28 = call "Plotting Convert XY to Waveform.vi"("Y"=dbl[] [], "X"=dbl[] []) -> ("Waveform Graph"=w71:waveform(dbl))  [unwired: 7 in, 2 out]
      n29 = call "Plotting Convert XY to Waveform.vi"("Y"=dbl[] [], "X"=dbl[] []) -> ("Waveform Graph"=w68:waveform(dbl))  [unwired: 7 in, 2 out]
      n30 = call "Plotting Convert XY to Waveform.vi"("Y"=dbl[] [], "X"=dbl[] []) -> ("Waveform Graph"=w65:waveform(dbl))  [unwired: 7 in, 2 out]
      n31 = call "Plotting Convert XY to Waveform.vi"("Y"=dbl[] [], "X"=dbl[] []) -> ("Waveform Graph"=w62:waveform(dbl))  [unwired: 7 in, 2 out]
      n32 = call "Plotting Convert XY to Waveform.vi"("Y"=dbl[] [], "X"=dbl[] []) -> ("Waveform Graph"=w59:waveform(dbl))  [unwired: 7 in, 2 out]
      n33 = call "Plotting Convert XY to Waveform.vi"("Y"=dbl[] [], "X"=dbl[] []) -> ("Waveform Graph"=w56:waveform(dbl))  [unwired: 7 in, 2 out]
      n34 = Bundle "Bundle"("Waveform Graph"=w88, "Waveform Graph"=w83, "Waveform Graph"=w77, "Waveform Graph"=w74, "Waveform Graph"=w71, "Waveform Graph"=w68, "Waveform Graph"=w65, "Waveform Graph"=w62, "Waveform Graph"=w59, "Waveform Graph"=w56) -> (w92:T1)  [unwired: 1 in]
    }
    frame 3 {
      n35 = Index Array(array=w133, index=0) -> (element=w93:i32)
      n36 = Index Array(array=w133, index=1) -> (element=w94:i32)
      n37 = Index Array(array=w133, index=2) -> (element=w95:i32)
      n38 = Index Array(array=w132, index (col)=w93) -> (element=w130:dbl[])  [unwired: 1 in]
      n39 = Index Array(array=w132, index (col)=w94) -> (element=w126:dbl[])  [unwired: 1 in]
      n40 = Index Array(array=w132, index (col)=w95) -> (element=w121:dbl[])  [unwired: 1 in]
      n41 = Index Array(array=w119, index=w93) -> (element=w127:string)
      n42 = Index Array(array=w119, index=w94) -> (element=w123:string)
      n43 = Index Array(array=w119, index=w95) -> (element=w117:string)
      n44 = call "Plotting Convert XY to Waveform.vi"("Plot Name"=w127, "Y"=w130, "X"=w122) -> ("Waveform Graph"=w129:waveform(dbl))  [unwired: 6 in, 2 out]
      n45 = call "Plotting Convert XY to Waveform.vi"("Plot Name"=w123, "Y"=w126, "X"=w122) -> ("Waveform Graph"=w125:waveform(dbl))  [unwired: 6 in, 2 out]
      n46 = call "Plotting Convert XY to Waveform.vi"("Plot Name"=w117, "Y"=w121, "X"=w122) -> ("Waveform Graph"=w120:waveform(dbl))  [unwired: 6 in, 2 out]
      n47 = call "Plotting Convert XY to Waveform.vi"("Y"=dbl[] [], "X"=dbl[] []) -> ("Waveform Graph"=w114:waveform(dbl))  [unwired: 7 in, 2 out]
      n48 = call "Plotting Convert XY to Waveform.vi"("Y"=dbl[] [], "X"=dbl[] []) -> ("Waveform Graph"=w111:waveform(dbl))  [unwired: 7 in, 2 out]
      n49 = call "Plotting Convert XY to Waveform.vi"("Y"=dbl[] [], "X"=dbl[] []) -> ("Waveform Graph"=w108:waveform(dbl))  [unwired: 7 in, 2 out]
      n50 = call "Plotting Convert XY to Waveform.vi"("Y"=dbl[] [], "X"=dbl[] []) -> ("Waveform Graph"=w105:waveform(dbl))  [unwired: 7 in, 2 out]
      n51 = call "Plotting Convert XY to Waveform.vi"("Y"=dbl[] [], "X"=dbl[] []) -> ("Waveform Graph"=w102:waveform(dbl))  [unwired: 7 in, 2 out]
      n52 = call "Plotting Convert XY to Waveform.vi"("Y"=dbl[] [], "X"=dbl[] []) -> ("Waveform Graph"=w99:waveform(dbl))  [unwired: 7 in, 2 out]
      n53 = call "Plotting Convert XY to Waveform.vi"("Y"=dbl[] [], "X"=dbl[] []) -> ("Waveform Graph"=w96:waveform(dbl))  [unwired: 7 in, 2 out]
      n54 = Bundle "Bundle"("Waveform Graph"=w129, "Waveform Graph"=w125, "Waveform Graph"=w120, "Waveform Graph"=w114, "Waveform Graph"=w111, "Waveform Graph"=w108, "Waveform Graph"=w105, "Waveform Graph"=w102, "Waveform Graph"=w99, "Waveform Graph"=w96) -> (w131:T1)  [unwired: 1 in]
    }
    frame 4 {
      n55 = Index Array(array=w176, index=0) -> (element=w137:i32)
      n56 = Index Array(array=w176, index=1) -> (element=w136:i32)
      n57 = Index Array(array=w176, index=2) -> (element=w135:i32)
      n58 = Index Array(array=w176, index=3) -> (element=w134:i32)
      n59 = Index Array(array=w175, index (col)=w137) -> (element=w173:dbl[])  [unwired: 1 in]
      n60 = Index Array(array=w175, index (col)=w136) -> (element=w171:dbl[])  [unwired: 1 in]
      n61 = Index Array(array=w175, index (col)=w135) -> (element=w165:dbl[])  [unwired: 1 in]
      n62 = Index Array(array=w175, index (col)=w134) -> (element=w160:dbl[])  [unwired: 1 in]
      n63 = Index Array(array=w158, index=w137) -> (element=w166:string)
      n64 = Index Array(array=w158, index=w136) -> (element=w168:string)
      n65 = Index Array(array=w158, index=w135) -> (element=w162:string)
      n66 = Index Array(array=w158, index=w134) -> (element=w156:string)
      n67 = call "Plotting Convert XY to Waveform.vi"("Plot Name"=w166, "Y"=w173, "X"=w161) -> ("Waveform Graph"=w172:waveform(dbl))  [unwired: 6 in, 2 out]
      n68 = call "Plotting Convert XY to Waveform.vi"("Plot Name"=w168, "Y"=w171, "X"=w161) -> ("Waveform Graph"=w170:waveform(dbl))  [unwired: 6 in, 2 out]
      n69 = call "Plotting Convert XY to Waveform.vi"("Plot Name"=w162, "Y"=w165, "X"=w161) -> ("Waveform Graph"=w164:waveform(dbl))  [unwired: 6 in, 2 out]
      n70 = call "Plotting Convert XY to Waveform.vi"("Plot Name"=w156, "Y"=w160, "X"=w161) -> ("Waveform Graph"=w157:waveform(dbl))  [unwired: 6 in, 2 out]
      n71 = call "Plotting Convert XY to Waveform.vi"("Y"=dbl[] [], "X"=dbl[] []) -> ("Waveform Graph"=w153:waveform(dbl))  [unwired: 7 in, 2 out]
      n72 = call "Plotting Convert XY to Waveform.vi"("Y"=dbl[] [], "X"=dbl[] []) -> ("Waveform Graph"=w150:waveform(dbl))  [unwired: 7 in, 2 out]
      n73 = call "Plotting Convert XY to Waveform.vi"("Y"=dbl[] [], "X"=dbl[] []) -> ("Waveform Graph"=w149:waveform(dbl))  [unwired: 7 in, 2 out]
      n74 = call "Plotting Convert XY to Waveform.vi"("Y"=dbl[] [], "X"=dbl[] []) -> ("Waveform Graph"=w144:waveform(dbl))  [unwired: 7 in, 2 out]
      n75 = call "Plotting Convert XY to Waveform.vi"("Y"=dbl[] [], "X"=dbl[] []) -> ("Waveform Graph"=w141:waveform(dbl))  [unwired: 7 in, 2 out]
      n76 = call "Plotting Convert XY to Waveform.vi"("Y"=dbl[] [], "X"=dbl[] []) -> ("Waveform Graph"=w138:waveform(dbl))  [unwired: 7 in, 2 out]
      n77 = Bundle "Bundle"("Waveform Graph"=w172, "Waveform Graph"=w170, "Waveform Graph"=w164, "Waveform Graph"=w157, "Waveform Graph"=w153, "Waveform Graph"=w150, "Waveform Graph"=w149, "Waveform Graph"=w144, "Waveform Graph"=w141, "Waveform Graph"=w138) -> (w174:T1)  [unwired: 1 in]
    }
    frame 5 {
      n78 = Index Array(array=w220, index=0) -> (element=w181:i32)
      n79 = Index Array(array=w220, index=1) -> (element=w180:i32)
      n80 = Index Array(array=w220, index=2) -> (element=w179:i32)
      n81 = Index Array(array=w220, index=3) -> (element=w178:i32)
      n82 = Index Array(array=w220, index=4) -> (element=w177:i32)
      n83 = Index Array(array=w219, index (col)=w181) -> (element=w218:dbl[])  [unwired: 1 in]
      n84 = Index Array(array=w219, index (col)=w180) -> (element=w215:dbl[])  [unwired: 1 in]
      n85 = Index Array(array=w219, index (col)=w179) -> (element=w210:dbl[])  [unwired: 1 in]
      n86 = Index Array(array=w219, index (col)=w178) -> (element=w206:dbl[])  [unwired: 1 in]
      n87 = Index Array(array=w219, index (col)=w177) -> (element=w201:dbl[])  [unwired: 1 in]
      n88 = Index Array(array=w199, index=w181) -> (element=w216:string)
      n89 = Index Array(array=w199, index=w180) -> (element=w213:string)
      n90 = Index Array(array=w199, index=w179) -> (element=w207:string)
      n91 = Index Array(array=w199, index=w178) -> (element=w203:string)
      n92 = Index Array(array=w199, index=w177) -> (element=w197:string)
      n93 = call "Plotting Convert XY to Waveform.vi"("Plot Name"=w216, "Y"=w218, "X"=w202) -> ("Waveform Graph"=w217:waveform(dbl))  [unwired: 6 in, 2 out]
      n94 = call "Plotting Convert XY to Waveform.vi"("Plot Name"=w213, "Y"=w215, "X"=w202) -> ("Waveform Graph"=w212:waveform(dbl))  [unwired: 6 in, 2 out]
      n95 = call "Plotting Convert XY to Waveform.vi"("Plot Name"=w207, "Y"=w210, "X"=w202) -> ("Waveform Graph"=w209:waveform(dbl))  [unwired: 6 in, 2 out]
      n96 = call "Plotting Convert XY to Waveform.vi"("Plot Name"=w203, "Y"=w206, "X"=w202) -> ("Waveform Graph"=w205:waveform(dbl))  [unwired: 6 in, 2 out]
      n97 = call "Plotting Convert XY to Waveform.vi"("Plot Name"=w197, "Y"=w201, "X"=w202) -> ("Waveform Graph"=w200:waveform(dbl))  [unwired: 6 in, 2 out]
      n98 = call "Plotting Convert XY to Waveform.vi"("Y"=dbl[] [], "X"=dbl[] []) -> ("Waveform Graph"=w194:waveform(dbl))  [unwired: 7 in, 2 out]
      n99 = call "Plotting Convert XY to Waveform.vi"("Y"=dbl[] [], "X"=dbl[] []) -> ("Waveform Graph"=w191:waveform(dbl))  [unwired: 7 in, 2 out]
      n100 = call "Plotting Convert XY to Waveform.vi"("Y"=dbl[] [], "X"=dbl[] []) -> ("Waveform Graph"=w188:waveform(dbl))  [unwired: 7 in, 2 out]
      n101 = call "Plotting Convert XY to Waveform.vi"("Y"=dbl[] [], "X"=dbl[] []) -> ("Waveform Graph"=w185:waveform(dbl))  [unwired: 7 in, 2 out]
      n102 = call "Plotting Convert XY to Waveform.vi"("Y"=dbl[] [], "X"=dbl[] []) -> ("Waveform Graph"=w182:waveform(dbl))  [unwired: 7 in, 2 out]
      n103 = Bundle "Bundle"("Waveform Graph"=w217, "Waveform Graph"=w212, "Waveform Graph"=w209, "Waveform Graph"=w205, "Waveform Graph"=w200, "Waveform Graph"=w194, "Waveform Graph"=w191, "Waveform Graph"=w188, "Waveform Graph"=w185, "Waveform Graph"=w182) -> (w221:T1)  [unwired: 1 in]
    }
    frame 6 {
      n104 = Index Array(array=w266, index=0) -> (element=w229:i32)
      n105 = Index Array(array=w266, index=1) -> (element=w228:i32)
      n106 = Index Array(array=w266, index=2) -> (element=w227:i32)
      n107 = Index Array(array=w266, index=3) -> (element=w226:i32)
      n108 = Index Array(array=w266, index=4) -> (element=w223:i32)
      n109 = Index Array(array=w266, index=5) -> (element=w225:i32)
      n110 = Index Array(array=w265, index (col)=w229) -> (element=w264:dbl[])  [unwired: 1 in]
      n111 = Index Array(array=w265, index (col)=w228) -> (element=w260:dbl[])  [unwired: 1 in]
      n112 = Index Array(array=w265, index (col)=w227) -> (element=w256:dbl[])  [unwired: 1 in]
      n113 = Index Array(array=w265, index (col)=w226) -> (element=w252:dbl[])  [unwired: 1 in]
      n114 = Index Array(array=w265, index (col)=w223) -> (element=w248:dbl[])  [unwired: 1 in]
      n115 = Index Array(array=w265, index (col)=w225) -> (element=w245:dbl[])  [unwired: 1 in]
      n116 = Index Array(array=w224, index=w229) -> (element=w261:string)
      n117 = Index Array(array=w224, index=w228) -> (element=w257:string)
      n118 = Index Array(array=w224, index=w227) -> (element=w253:string)
      n119 = Index Array(array=w224, index=w226) -> (element=w249:string)
      n120 = Index Array(array=w224, index=w223) -> (element=w222:string)
      n121 = Index Array(array=w224, index=w225) -> (element=w242:string)
      n122 = call "Plotting Convert XY to Waveform.vi"("Plot Name"=w261, "Y"=w264, "X"=w246) -> ("Waveform Graph"=w263:waveform(dbl))  [unwired: 6 in, 2 out]
      n123 = call "Plotting Convert XY to Waveform.vi"("Plot Name"=w257, "Y"=w260, "X"=w246) -> ("Waveform Graph"=w259:waveform(dbl))  [unwired: 6 in, 2 out]
      n124 = call "Plotting Convert XY to Waveform.vi"("Plot Name"=w253, "Y"=w256, "X"=w246) -> ("Waveform Graph"=w255:waveform(dbl))  [unwired: 6 in, 2 out]
      n125 = call "Plotting Convert XY to Waveform.vi"("Plot Name"=w249, "Y"=w252, "X"=w246) -> ("Waveform Graph"=w251:waveform(dbl))  [unwired: 6 in, 2 out]
      n126 = call "Plotting Convert XY to Waveform.vi"("Plot Name"=w222, "Y"=w248, "X"=w246) -> ("Waveform Graph"=w247:waveform(dbl))  [unwired: 6 in, 2 out]
      n127 = call "Plotting Convert XY to Waveform.vi"("Plot Name"=w242, "Y"=w245, "X"=w246) -> ("Waveform Graph"=w244:waveform(dbl))  [unwired: 6 in, 2 out]
      n128 = call "Plotting Convert XY to Waveform.vi"("Y"=dbl[] [], "X"=dbl[] []) -> ("Waveform Graph"=w239:waveform(dbl))  [unwired: 7 in, 2 out]
      n129 = call "Plotting Convert XY to Waveform.vi"("Y"=dbl[] [], "X"=dbl[] []) -> ("Waveform Graph"=w238:waveform(dbl))  [unwired: 7 in, 2 out]
      n130 = call "Plotting Convert XY to Waveform.vi"("Y"=dbl[] [], "X"=dbl[] []) -> ("Waveform Graph"=w235:waveform(dbl))  [unwired: 7 in, 2 out]
      n131 = call "Plotting Convert XY to Waveform.vi"("Y"=dbl[] [], "X"=dbl[] []) -> ("Waveform Graph"=w230:waveform(dbl))  [unwired: 7 in, 2 out]
      n132 = Bundle "Bundle"("Waveform Graph"=w263, "Waveform Graph"=w259, "Waveform Graph"=w255, "Waveform Graph"=w251, "Waveform Graph"=w247, "Waveform Graph"=w244, "Waveform Graph"=w239, "Waveform Graph"=w238, "Waveform Graph"=w235, "Waveform Graph"=w230) -> (w267:T1)  [unwired: 1 in]
    }
    frame 7 {
      n133 = Index Array(array=w317, index=0) -> (element=w269:i32)
      n134 = Index Array(array=w317, index=1) -> (element=w270:i32)
      n135 = Index Array(array=w317, index=2) -> (element=w271:i32)
      n136 = Index Array(array=w317, index=3) -> (element=w272:i32)
      n137 = Index Array(array=w317, index=4) -> (element=w273:i32)
      n138 = Index Array(array=w317, index=5) -> (element=w274:i32)
      n139 = Index Array(array=w317, index=6) -> (element=w275:i32)
      n140 = Index Array(array=w316, index (col)=w269) -> (element=w314:dbl[])  [unwired: 1 in]
      n141 = Index Array(array=w316, index (col)=w270) -> (element=w312:dbl[])  [unwired: 1 in]
      n142 = Index Array(array=w316, index (col)=w271) -> (element=w306:dbl[])  [unwired: 1 in]
      n143 = Index Array(array=w316, index (col)=w272) -> (element=w302:dbl[])  [unwired: 1 in]
      n144 = Index Array(array=w316, index (col)=w273) -> (element=w298:dbl[])  [unwired: 1 in]
      n145 = Index Array(array=w316, index (col)=w274) -> (element=w294:dbl[])  [unwired: 1 in]
      n146 = Index Array(array=w316, index (col)=w275) -> (element=w289:dbl[])  [unwired: 1 in]
      n147 = Index Array(array=w287, index=w269) -> (element=w309:string)
      n148 = Index Array(array=w287, index=w270) -> (element=w307:string)
      n149 = Index Array(array=w287, index=w271) -> (element=w303:string)
      n150 = Index Array(array=w287, index=w272) -> (element=w299:string)
      n151 = Index Array(array=w287, index=w273) -> (element=w295:string)
      n152 = Index Array(array=w287, index=w274) -> (element=w291:string)
      n153 = Index Array(array=w287, index=w275) -> (element=w285:string)
      n154 = call "Plotting Convert XY to Waveform.vi"("Plot Name"=w309, "Y"=w314, "X"=w290) -> ("Waveform Graph"=w313:waveform(dbl))  [unwired: 6 in, 2 out]
      n155 = call "Plotting Convert XY to Waveform.vi"("Plot Name"=w307, "Y"=w312, "X"=w290) -> ("Waveform Graph"=w311:waveform(dbl))  [unwired: 6 in, 2 out]
      n156 = call "Plotting Convert XY to Waveform.vi"("Plot Name"=w303, "Y"=w306, "X"=w290) -> ("Waveform Graph"=w305:waveform(dbl))  [unwired: 6 in, 2 out]
      n157 = call "Plotting Convert XY to Waveform.vi"("Plot Name"=w299, "Y"=w302, "X"=w290) -> ("Waveform Graph"=w301:waveform(dbl))  [unwired: 6 in, 2 out]
      n158 = call "Plotting Convert XY to Waveform.vi"("Plot Name"=w295, "Y"=w298, "X"=w290) -> ("Waveform Graph"=w297:waveform(dbl))  [unwired: 6 in, 2 out]
      n159 = call "Plotting Convert XY to Waveform.vi"("Plot Name"=w291, "Y"=w294, "X"=w290) -> ("Waveform Graph"=w293:waveform(dbl))  [unwired: 6 in, 2 out]
      n160 = call "Plotting Convert XY to Waveform.vi"("Plot Name"=w285, "Y"=w289, "X"=w290) -> ("Waveform Graph"=w288:waveform(dbl))  [unwired: 6 in, 2 out]
      n161 = call "Plotting Convert XY to Waveform.vi"("Y"=dbl[] [], "X"=dbl[] []) -> ("Waveform Graph"=w282:waveform(dbl))  [unwired: 7 in, 2 out]
      n162 = call "Plotting Convert XY to Waveform.vi"("Y"=dbl[] [], "X"=dbl[] []) -> ("Waveform Graph"=w279:waveform(dbl))  [unwired: 7 in, 2 out]
      n163 = call "Plotting Convert XY to Waveform.vi"("Y"=dbl[] [], "X"=dbl[] []) -> ("Waveform Graph"=w276:waveform(dbl))  [unwired: 7 in, 2 out]
      n164 = Bundle "Bundle"("Waveform Graph"=w313, "Waveform Graph"=w311, "Waveform Graph"=w305, "Waveform Graph"=w301, "Waveform Graph"=w297, "Waveform Graph"=w293, "Waveform Graph"=w288, "Waveform Graph"=w282, "Waveform Graph"=w279, "Waveform Graph"=w276) -> (w315:T1)  [unwired: 1 in]
    }
    frame 8 {
      n165 = Index Array(array=w367, index=0) -> (element=w320:i32)
      n166 = Index Array(array=w367, index=1) -> (element=w321:i32)
      n167 = Index Array(array=w367, index=2) -> (element=w322:i32)
      n168 = Index Array(array=w367, index=3) -> (element=w323:i32)
      n169 = Index Array(array=w367, index=4) -> (element=w324:i32)
      n170 = Index Array(array=w367, index=5) -> (element=w325:i32)
      n171 = Index Array(array=w367, index=6) -> (element=w326:i32)
      n172 = Index Array(array=w367, index=7) -> (element=w327:i32)
      n173 = Index Array(array=w366, index (col)=w320) -> (element=w318:dbl[])  [unwired: 1 in]
      n174 = Index Array(array=w366, index (col)=w321) -> (element=w362:dbl[])  [unwired: 1 in]
      n175 = Index Array(array=w366, index (col)=w322) -> (element=w358:dbl[])  [unwired: 1 in]
      n176 = Index Array(array=w366, index (col)=w323) -> (element=w354:dbl[])  [unwired: 1 in]
      n177 = Index Array(array=w366, index (col)=w324) -> (element=w350:dbl[])  [unwired: 1 in]
      n178 = Index Array(array=w366, index (col)=w325) -> (element=w346:dbl[])  [unwired: 1 in]
      n179 = Index Array(array=w366, index (col)=w326) -> (element=w342:dbl[])  [unwired: 1 in]
      n180 = Index Array(array=w366, index (col)=w327) -> (element=w338:dbl[])  [unwired: 1 in]
      n181 = Index Array(array=w335, index=w320) -> (element=w363:string)
      n182 = Index Array(array=w335, index=w321) -> (element=w359:string)
      n183 = Index Array(array=w335, index=w322) -> (element=w355:string)
      n184 = Index Array(array=w335, index=w323) -> (element=w351:string)
      n185 = Index Array(array=w335, index=w324) -> (element=w347:string)
      n186 = Index Array(array=w335, index=w325) -> (element=w343:string)
      n187 = Index Array(array=w335, index=w326) -> (element=w339:string)
      n188 = Index Array(array=w335, index=w327) -> (element=w334:string)
      n189 = call "Plotting Convert XY to Waveform.vi"("Plot Name"=w363, "Y"=w318, "X"=w319) -> ("Waveform Graph"=w364:waveform(dbl))  [unwired: 6 in, 2 out]
      n190 = call "Plotting Convert XY to Waveform.vi"("Plot Name"=w359, "Y"=w362, "X"=w319) -> ("Waveform Graph"=w361:waveform(dbl))  [unwired: 6 in, 2 out]
      n191 = call "Plotting Convert XY to Waveform.vi"("Plot Name"=w355, "Y"=w358, "X"=w319) -> ("Waveform Graph"=w357:waveform(dbl))  [unwired: 6 in, 2 out]
      n192 = call "Plotting Convert XY to Waveform.vi"("Plot Name"=w351, "Y"=w354, "X"=w319) -> ("Waveform Graph"=w353:waveform(dbl))  [unwired: 6 in, 2 out]
      n193 = call "Plotting Convert XY to Waveform.vi"("Plot Name"=w347, "Y"=w350, "X"=w319) -> ("Waveform Graph"=w349:waveform(dbl))  [unwired: 6 in, 2 out]
      n194 = call "Plotting Convert XY to Waveform.vi"("Plot Name"=w343, "Y"=w346, "X"=w319) -> ("Waveform Graph"=w345:waveform(dbl))  [unwired: 6 in, 2 out]
      n195 = call "Plotting Convert XY to Waveform.vi"("Plot Name"=w339, "Y"=w342, "X"=w319) -> ("Waveform Graph"=w341:waveform(dbl))  [unwired: 6 in, 2 out]
      n196 = call "Plotting Convert XY to Waveform.vi"("Plot Name"=w334, "Y"=w338, "X"=w319) -> ("Waveform Graph"=w337:waveform(dbl))  [unwired: 6 in, 2 out]
      n197 = call "Plotting Convert XY to Waveform.vi"("Y"=dbl[] [], "X"=dbl[] []) -> ("Waveform Graph"=w331:waveform(dbl))  [unwired: 7 in, 2 out]
      n198 = call "Plotting Convert XY to Waveform.vi"("Y"=dbl[] [], "X"=dbl[] []) -> ("Waveform Graph"=w328:waveform(dbl))  [unwired: 7 in, 2 out]
      n199 = Bundle "Bundle"("Waveform Graph"=w364, "Waveform Graph"=w361, "Waveform Graph"=w357, "Waveform Graph"=w353, "Waveform Graph"=w349, "Waveform Graph"=w345, "Waveform Graph"=w341, "Waveform Graph"=w337, "Waveform Graph"=w331, "Waveform Graph"=w328) -> (w368:T1)  [unwired: 1 in]
    }
    frame 9 {
      n200 = Index Array(array=w421, index=0) -> (element=w369:i32)
      n201 = Index Array(array=w421, index=1) -> (element=w370:i32)
      n202 = Index Array(array=w421, index=2) -> (element=w371:i32)
      n203 = Index Array(array=w421, index=3) -> (element=w372:i32)
      n204 = Index Array(array=w421, index=4) -> (element=w374:i32)
      n205 = Index Array(array=w421, index=5) -> (element=w375:i32)
      n206 = Index Array(array=w421, index=6) -> (element=w376:i32)
      n207 = Index Array(array=w421, index=7) -> (element=w377:i32)
      n208 = Index Array(array=w421, index=8) -> (element=w378:i32)
      n209 = Index Array(array=w420, index (col)=w369) -> (element=w418:dbl[])  [unwired: 1 in]
      n210 = Index Array(array=w420, index (col)=w370) -> (element=w416:dbl[])  [unwired: 1 in]
      n211 = Index Array(array=w420, index (col)=w371) -> (element=w410:dbl[])  [unwired: 1 in]
      n212 = Index Array(array=w420, index (col)=w372) -> (element=w406:dbl[])  [unwired: 1 in]
      n213 = Index Array(array=w420, index (col)=w374) -> (element=w402:dbl[])  [unwired: 1 in]
      n214 = Index Array(array=w420, index (col)=w375) -> (element=w399:dbl[])  [unwired: 1 in]
      n215 = Index Array(array=w420, index (col)=w376) -> (element=w395:dbl[])  [unwired: 1 in]
      n216 = Index Array(array=w420, index (col)=w377) -> (element=w390:dbl[])  [unwired: 1 in]
      n217 = Index Array(array=w420, index (col)=w378) -> (element=w387:dbl[])  [unwired: 1 in]
      n218 = Index Array(array=w385, index=w369) -> (element=w413:string)
      n219 = Index Array(array=w385, index=w370) -> (element=w411:string)
      n220 = Index Array(array=w385, index=w371) -> (element=w407:string)
      n221 = Index Array(array=w385, index=w372) -> (element=w404:string)
      n222 = Index Array(array=w385, index=w374) -> (element=w400:string)
      n223 = Index Array(array=w385, index=w375) -> (element=w396:string)
      n224 = Index Array(array=w385, index=w376) -> (element=w392:string)
      n225 = Index Array(array=w385, index=w377) -> (element=w379:string)
      n226 = Index Array(array=w385, index=w378) -> (element=w383:string)
      n227 = call "Plotting Convert XY to Waveform.vi"("Plot Name"=w413, "Y"=w418, "X"=w388) -> ("Waveform Graph"=w417:waveform(dbl))  [unwired: 6 in, 2 out]
      n228 = call "Plotting Convert XY to Waveform.vi"("Plot Name"=w411, "Y"=w416, "X"=w388) -> ("Waveform Graph"=w415:waveform(dbl))  [unwired: 6 in, 2 out]
      n229 = call "Plotting Convert XY to Waveform.vi"("Plot Name"=w407, "Y"=w410, "X"=w388) -> ("Waveform Graph"=w409:waveform(dbl))  [unwired: 6 in, 2 out]
      n230 = call "Plotting Convert XY to Waveform.vi"("Plot Name"=w404, "Y"=w406, "X"=w388) -> ("Waveform Graph"=w405:waveform(dbl))  [unwired: 6 in, 2 out]
      n231 = call "Plotting Convert XY to Waveform.vi"("Plot Name"=w400, "Y"=w402, "X"=w388) -> ("Waveform Graph"=w401:waveform(dbl))  [unwired: 6 in, 2 out]
      n232 = call "Plotting Convert XY to Waveform.vi"("Plot Name"=w396, "Y"=w399, "X"=w388) -> ("Waveform Graph"=w398:waveform(dbl))  [unwired: 6 in, 2 out]
      n233 = call "Plotting Convert XY to Waveform.vi"("Plot Name"=w392, "Y"=w395, "X"=w388) -> ("Waveform Graph"=w394:waveform(dbl))  [unwired: 6 in, 2 out]
      n234 = call "Plotting Convert XY to Waveform.vi"("Plot Name"=w379, "Y"=w390, "X"=w388) -> ("Waveform Graph"=w389:waveform(dbl))  [unwired: 6 in, 2 out]
      n235 = call "Plotting Convert XY to Waveform.vi"("Plot Name"=w383, "Y"=w387, "X"=w388) -> ("Waveform Graph"=w386:waveform(dbl))  [unwired: 6 in, 2 out]
      n236 = call "Plotting Convert XY to Waveform.vi"("Y"=dbl[] [], "X"=dbl[] []) -> ("Waveform Graph"=w380:waveform(dbl))  [unwired: 7 in, 2 out]
      n237 = Bundle "Bundle"("Waveform Graph"=w417, "Waveform Graph"=w415, "Waveform Graph"=w409, "Waveform Graph"=w405, "Waveform Graph"=w401, "Waveform Graph"=w398, "Waveform Graph"=w394, "Waveform Graph"=w389, "Waveform Graph"=w386, "Waveform Graph"=w380) -> (w419:T1)  [unwired: 1 in]
    }
    frame 10 {
      n238 = Index Array(array=w473, index=0) -> (element=w422:i32)
      n239 = Index Array(array=w473, index=1) -> (element=w423:i32)
      n240 = Index Array(array=w473, index=2) -> (element=w424:i32)
      n241 = Index Array(array=w473, index=3) -> (element=w425:i32)
      n242 = Index Array(array=w473, index=4) -> (element=w426:i32)
      n243 = Index Array(array=w473, index=5) -> (element=w427:i32)
      n244 = Index Array(array=w473, index=6) -> (element=w428:i32)
      n245 = Index Array(array=w473, index=7) -> (element=w429:i32)
      n246 = Index Array(array=w473, index=8) -> (element=w430:i32)
      n247 = Index Array(array=w473, index=9) -> (element=w431:i32)
      n248 = Index Array(array=w476, index (col)=w422) -> (element=w475:dbl[])  [unwired: 1 in]
      n249 = Index Array(array=w476, index (col)=w423) -> (element=w469:dbl[])  [unwired: 1 in]
      n250 = Index Array(array=w476, index (col)=w424) -> (element=w466:dbl[])  [unwired: 1 in]
      n251 = Index Array(array=w476, index (col)=w425) -> (element=w462:dbl[])  [unwired: 1 in]
      n252 = Index Array(array=w476, index (col)=w426) -> (element=w458:dbl[])  [unwired: 1 in]
      n253 = Index Array(array=w476, index (col)=w427) -> (element=w454:dbl[])  [unwired: 1 in]
      n254 = Index Array(array=w476, index (col)=w428) -> (element=w450:dbl[])  [unwired: 1 in]
      n255 = Index Array(array=w476, index (col)=w429) -> (element=w446:dbl[])  [unwired: 1 in]
      n256 = Index Array(array=w476, index (col)=w430) -> (element=w442:dbl[])  [unwired: 1 in]
      n257 = Index Array(array=w476, index (col)=w431) -> (element=w435:dbl[])  [unwired: 1 in]
      n258 = Index Array(array=w437, index=w422) -> (element=w471:string)
      n259 = Index Array(array=w437, index=w423) -> (element=w467:string)
      n260 = Index Array(array=w437, index=w424) -> (element=w463:string)
      n261 = Index Array(array=w437, index=w425) -> (element=w459:string)
      n262 = Index Array(array=w437, index=w426) -> (element=w455:string)
      n263 = Index Array(array=w437, index=w427) -> (element=w451:string)
      n264 = Index Array(array=w437, index=w428) -> (element=w447:string)
      n265 = Index Array(array=w437, index=w429) -> (element=w443:string)
      n266 = Index Array(array=w437, index=w430) -> (element=w439:string)
      n267 = Index Array(array=w437, index=w431) -> (element=w433:string)
      n268 = call "Plotting Convert XY to Waveform.vi"("Plot Name"=w471, "Y"=w475, "X"=w436) -> ("Waveform Graph"=w474:waveform(dbl))  [unwired: 6 in, 2 out]
      n269 = call "Plotting Convert XY to Waveform.vi"("Plot Name"=w467, "Y"=w469, "X"=w436) -> ("Waveform Graph"=w468:waveform(dbl))  [unwired: 6 in, 2 out]
      n270 = call "Plotting Convert XY to Waveform.vi"("Plot Name"=w463, "Y"=w466, "X"=w436) -> ("Waveform Graph"=w465:waveform(dbl))  [unwired: 6 in, 2 out]
      n271 = call "Plotting Convert XY to Waveform.vi"("Plot Name"=w459, "Y"=w462, "X"=w436) -> ("Waveform Graph"=w461:waveform(dbl))  [unwired: 6 in, 2 out]
      n272 = call "Plotting Convert XY to Waveform.vi"("Plot Name"=w455, "Y"=w458, "X"=w436) -> ("Waveform Graph"=w457:waveform(dbl))  [unwired: 6 in, 2 out]
      n273 = call "Plotting Convert XY to Waveform.vi"("Plot Name"=w451, "Y"=w454, "X"=w436) -> ("Waveform Graph"=w453:waveform(dbl))  [unwired: 6 in, 2 out]
      n274 = call "Plotting Convert XY to Waveform.vi"("Plot Name"=w447, "Y"=w450, "X"=w436) -> ("Waveform Graph"=w449:waveform(dbl))  [unwired: 6 in, 2 out]
      n275 = call "Plotting Convert XY to Waveform.vi"("Plot Name"=w443, "Y"=w446, "X"=w436) -> ("Waveform Graph"=w445:waveform(dbl))  [unwired: 6 in, 2 out]
      n276 = call "Plotting Convert XY to Waveform.vi"("Plot Name"=w439, "Y"=w442, "X"=w436) -> ("Waveform Graph"=w441:waveform(dbl))  [unwired: 6 in, 2 out]
      n277 = call "Plotting Convert XY to Waveform.vi"("Plot Name"=w433, "Y"=w435, "X"=w436) -> ("Waveform Graph"=w434:waveform(dbl))  [unwired: 6 in, 2 out]
      n278 = Bundle "Bundle"("Waveform Graph"=w474, "Waveform Graph"=w468, "Waveform Graph"=w465, "Waveform Graph"=w461, "Waveform Graph"=w457, "Waveform Graph"=w453, "Waveform Graph"=w449, "Waveform Graph"=w445, "Waveform Graph"=w441, "Waveform Graph"=w434) -> (w432:T1)  [unwired: 1 in]
    }
  }
  "Mixed Signal Graph" <- w10
  "Error Out" <- "Error In"
